vi "SetParam.vi"(8 "error in (no error)":errorcluster caption="entrée d'erreur (pas d'erreur)", 10 "maxabs_scale":cluster{"axis":i32, "copy":bool}={"axis"=0, "copy"=TRUE}, 11 "maxabs_scale.lvclass":refnum<class "maxabs_scale.lvclass">) -> (0 "error out":errorcluster caption="sortie d'erreur", 3 "maxabs_scale.lvclass":refnum<class "maxabs_scale.lvclass">)   [LabVIEW 2020, in "maxabs_scale.lvclass"]
doc: "Set Parameters"
uses:
  maxabs_scale.lvclass
  maxabs_scale.lvclass/maxabs_scale.ctl
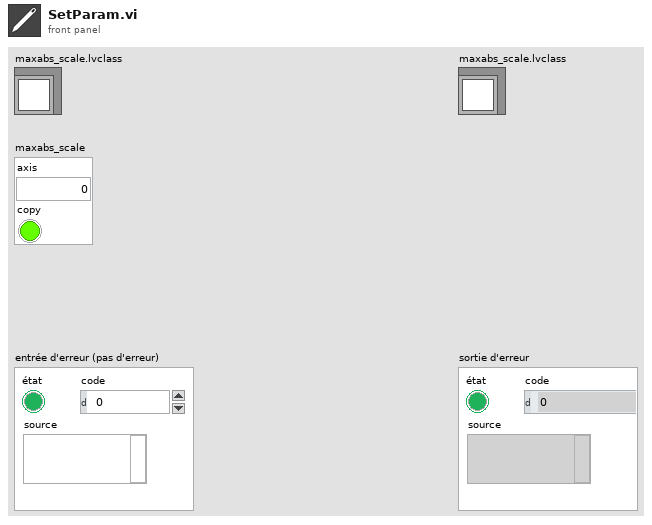
[diagram p1: front panel]
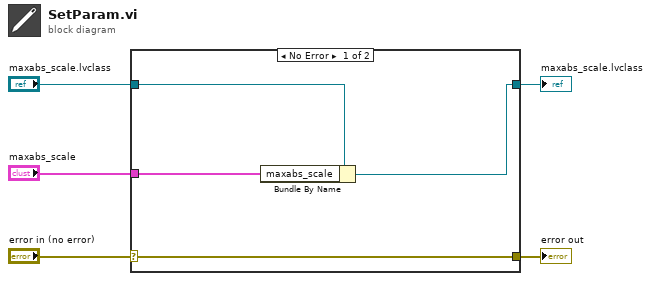
[diagram p0: block diagram]
diagram:
  n1 = case shown="No Error" "error in (no error)" {
    selector: "error in (no error)" -> [w9 w10]
    tunnel: [w9 w10] -> w4
    tunnel: [w7 w11] -> w2
    tunnel: "maxabs_scale.lvclass" -> [w8 w11]
    tunnel: "maxabs_scale" -> [w6 _]
    frame No Error {
      n2 = Bundle By Name(cluster=w8, "maxabs_scale"=w6) -> (w7:refnum<class "maxabs_scale.lvclass">)
    }
    frame Error {
    }
  }
  "error out" <- w4
  "maxabs_scale.lvclass" <- w2
